vi "GitSave.vi"(4 "Date":string, 6 "Commit Meta-Info":T3, 7 "Make LAST_SAVED":bool=TRUE, 8 "error in (no error)":errorcluster, 9 "Save Repo Path":path=path "", 10 "Save Cluster":T1 {"Select Layout" items=["Default"]}, 11 "Git exec":string="git") -> (0 "error out":errorcluster, 1 "User Cancelled":bool, 2 "Saved Hash":string, 3 "Git exec out":string="git")   [LabVIEW 2013]
uses:
  TypeDefs/SaveCluster.ctl
  VariableManagerCodes/VariableManager/VariableManager.lvclass
  DeviceVIs/Device/Device.lvclass
  <vilib>/Utility/miscctls.llb/LVStringsAndValuesArrayTypeDef_I32.ctl
  <vilib>/Utility/error.llb/DialogType.ctl
panel:
  out "Response":string
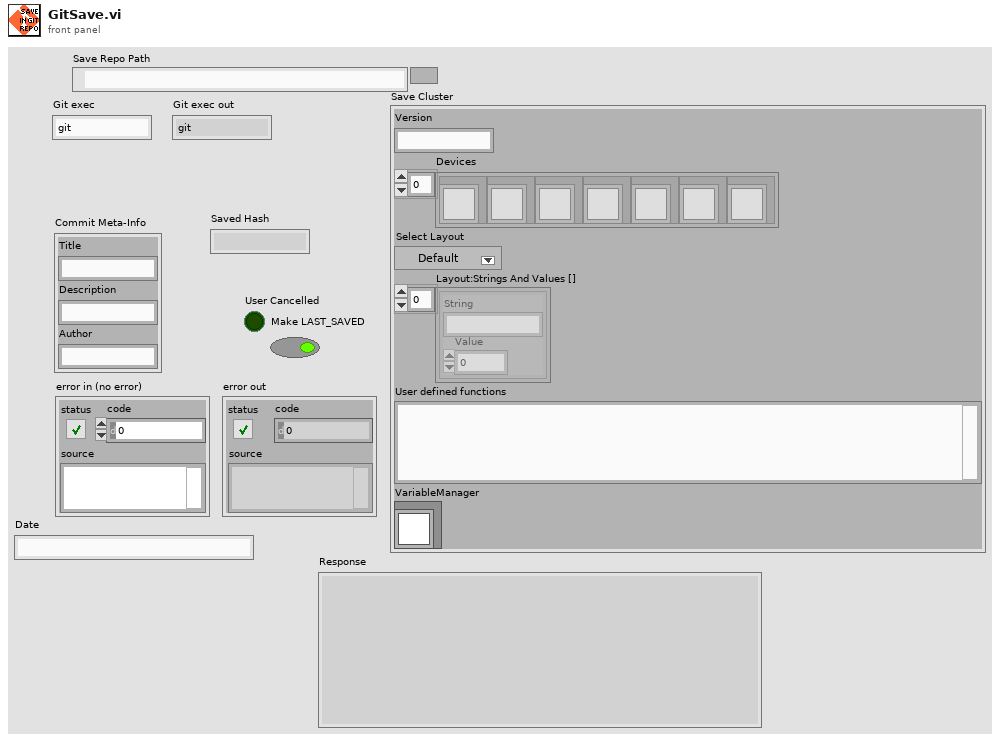
[diagram p1: front panel]
types:
  T1 = typedef "SaveCluster.ctl" = cluster{"Version":string, "Devices":refnum<class "Device.lvclass">[], "Select Layout":i32, "Layout:Strings And Values []":T2, "User defined functions":string, "VariableManager":refnum<class "VariableManager.lvclass">}
  T2 = typedef "LVStringsAndValuesArrayTypeDef_I32.ctl" = cluster{"String":string, "Value":i32}[]
  T3 = cluster{"Title":string, "Description":string, "Author":string}
  T4 = typedef "DialogType.ctl" = u16
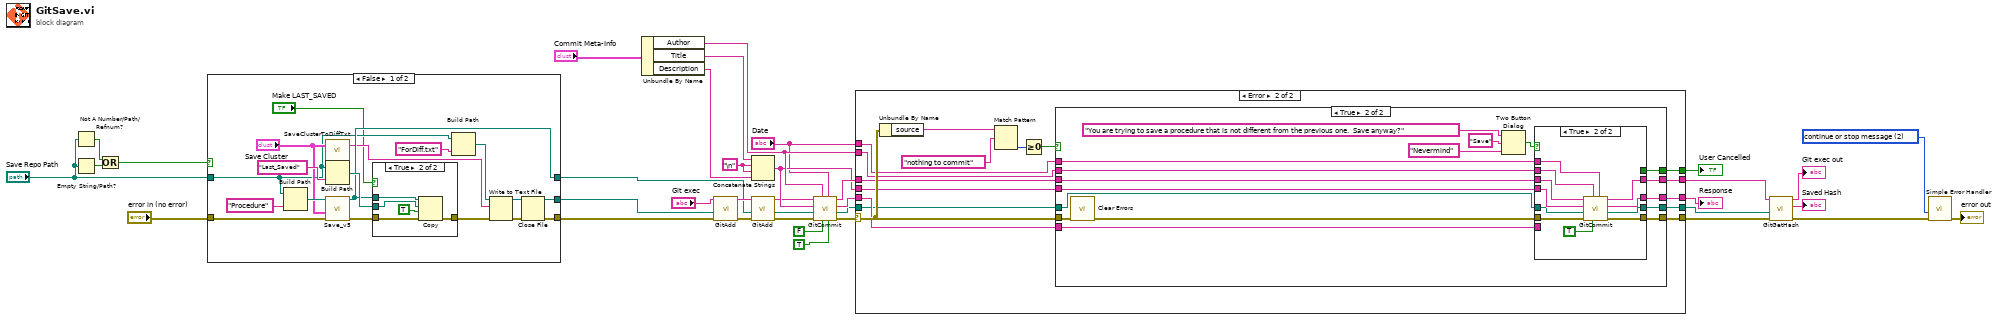
[diagram p0: block diagram]
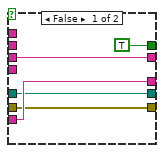
[diagram p6: hidden frame]
diagram:
  w1 = T4 2 items=["no dialog", "OK message", "continue or stop message", "OK message + warnings", "continue/stop + warnings"] ("type of dialog (OK msg:1)")
  w32 = "\n"
  n1 = Not A Number/Path/Refnum?(number/path/refnum="Save Repo Path") -> (NaN/Path/Refnum?=w14:bool)
  n2 = Empty String/Path?(string/path="Save Repo Path") -> (empty?=w13:bool)
  n3 = Or(x=w14, y=w13) -> (x .or. y?=w12:bool)
  n4 = case shown="False" w12 {
    tunnel: "error in (no error)" -> [w55 w63]
    tunnel: [w40 w63] -> w36
    tunnel: [w49 w62] -> w5
    tunnel: "Save Repo Path" -> [w44 w62]
    tunnel: [w39 w62] -> w6
    frame False {
      n5 = Build Path(base path=w44, name or relative path="Procedure") -> (appended path=w52:path)
      n6 = call "SaveClusterToDiffTxt.vi"("Save Cluster"="Save Cluster") -> ("DiffText"=w46:string)  [unwired: 2 in]
      n7 = Build Path(base path=w44, name or relative path="Last_Saved") -> (appended path=w51:path)
      n8 = call "Save_v5.vi"("error in"=w55, "Save Cluster"="Save Cluster", "Path (open dialog)"=w52) -> ("error out"=w50:errorcluster, "Chosen Path"=w49:path)  [unwired: 5 in, 2 out]
      n9 = case shown="True" "Make LAST_SAVED" {
        tunnel: w51 -> [_ w61]
        tunnel: w50 -> [w56 w59]
        tunnel: w49 -> [_ w58]
        tunnel: [w56 w57] -> w45
        frame False {
        }
        frame True {
          n10 = Copy(8:w59, 9:TRUE ("overwrite (F)"), 10:w61, 11:w58) -> (0:w57:errorcluster)  [unwired: 1 in, 2 out]
        }
      }
      n11 = Build Path(base path=w44, name or relative path="ForDiff.txt") -> (appended path=w43:path)
      n12 = Write to Text File(file (use dialog)=w43, text=w46, error in=w45) -> (refnum out=w41:refnum<file>, error out=w42:errorcluster)  [unwired: 1 in, 1 out]
      n13 = Close File(refnum=w41, error in=w42) -> (path=w39:path, error out=w40:errorcluster)
    }
    frame True {
    }
  }
  n14 = Unbundle By Name("Commit Meta-Info") -> ("Author"=w19:string, "Title"=w34:string, "Description"=w33:string)
  n15 = call "GitAdd.vi"("error in (no error)"=w36, "File"=w6, "Git exec"="Git exec") -> ("error out"=w10:errorcluster, "Git exec out"=w11:string)  [unwired: 5 in, 2 out]
  n16 = Concatenate Strings(w34, w32, w32, w33) -> (w18:string)
  n17 = call "GitAdd.vi"("error in (no error)"=w10, "File"=w5, "Git exec"=w11) -> ("error out"=w9:errorcluster, "File out"=w7:path, "Git exec out"=w8:string)  [unwired: 5 in, 1 out]
  n18 = call "GitCommit.vi"("CommitAllAdded"=TRUE, "Date"="Date", "Allow Empty Commit?"=FALSE, "Author"=w19, "error in (no error)"=w9, "File"=w7, "Commit Message"=w18, "Git exec"=w8) -> ("error out"=w27:errorcluster, "File out"=w21:path, "Response"=w23:string, "Git exec out"=w25:string)
  n19 = case shown="Error" w27 {
    selector: w27 -> [w67 w79]
    tunnel: [w67 w78] -> w26
    tunnel: w25 -> [w66 w77]
    tunnel: [w66 w72] -> w24
    tunnel: w23 -> [w65 w76]
    tunnel: [w65 w73] -> w22
    tunnel: w21 -> [w64 w75]
    tunnel: [w64 w74] -> w20
    tunnel: w19 -> [_ w71]
    tunnel: w18 -> [_ w70]
    tunnel: [_ w69] -> w17
    tunnel: "Date" -> [_ w68]
    frame No Error {
    }
    frame Error {
      n20 = Unbundle By Name(w79) -> ("source"=w83:string)
      n21 = Match Pattern(string=w83, regular expression="nothing to commit") -> (offset past match=w81:i32)  [unwired: 1 in, 3 out]
      n22 = Greater Or Equal To 0?(x=w81) -> (x >= 0?=w80:bool)
      n23 = case shown="True" w80 {
        tunnel: w79 -> [w87 w100]
        tunnel: [w87 w99] -> w78
        tunnel: w77 -> [w84 w93]
        tunnel: w76 -> [w85 w90]
        tunnel: w75 -> [w86 w91]
        tunnel: [w86 w98] -> w74
        tunnel: [w85 w97] -> w73
        tunnel: [w84 w96] -> w72
        tunnel: w71 -> [_ w95]
        tunnel: w70 -> [_ w94]
        tunnel: [_ w89] -> w69
        tunnel: w68 -> [_ w88]
        frame False {
        }
        frame True {
          n24 = call <vilib>:"Clear Errors.vi"("error in (no error)"=w100) -> ("error out"=w92:errorcluster)  [unwired: 6 in]
          n25 = Two Button Dialog(message="You are trying to save a procedure that is not different from the previous one.  Save anyway?", 1:"Nevermind" ("F button name (\"Cancel\")"), 2:"Save" ("T button name (\"OK\")")) -> (T button?=w101:bool)
          n26 = case shown="True" w101 {
            tunnel: [w108 w120] -> w99
            tunnel: [w107 w119] -> w98
            tunnel: [w109 w118] -> w97
            tunnel: [w106 w117] -> w96
            tunnel: w95 -> [_ w116]
            tunnel: w94 -> [_ w115]
            tunnel: w93 -> [w106 w114]
            tunnel: w92 -> [w108 w113]
            tunnel: w91 -> [w107 w112]
            tunnel: w90 -> [w109 _]
            tunnel: [TRUE _] -> w89
            tunnel: w88 -> [_ w110]
            frame False {
            }
            frame True {
              n27 = call "GitCommit.vi"("Date"=w110, "Allow Empty Commit?"=TRUE, "Author"=w116, "error in (no error)"=w113, "File"=w112, "Commit Message"=w115, "Git exec"=w114) -> ("error out"=w120:errorcluster, "File out"=w119:path, "Response"=w118:string, "Git exec out"=w117:string)  [unwired: 1 in]
            }
          }
        }
      }
    }
  }
  "Response" <- w22
  "User Cancelled" <- w17
  n28 = call "GitGetHash.vi"("error in (no error)"=w26, "Directory"=w20, "Git exec"=w24) -> ("error out"=w3:errorcluster, "Hash"=→"Saved Hash":string, "Git exec out"=→"Git exec out":string)  [unwired: 5 in, 1 out]
  n29 = call <vilib>:"Simple Error Handler.vi"("type of dialog (OK msg:1)"=w1, "error in (no error)"=w3) -> ("error out"=→"error out":errorcluster)  [unwired: 3 in, 4 out]
